vi "DFU_Foot_Data.vi"() -> ()   [LabVIEW 2016]
uses:
  <vilib>/Math Plots/3D Math Plots/3D Surface/3D Surface XCtrl/3D Surface.xctl
  <vilib>/Math Plots/3D Math Plots/3D Surface/3D Surface Datatype/Public/Plot Helper (Matrix).vi
  <vilib>/gmath/interp.llb/Interpolate 2D (2d X,Y).vi
  <vilib>/Math Plots/3D Math Plots/3D Surface/3D Surface Datatype/3D Surface Datatype.lvclass
  <vilib>/gmath/NI_Gmath.lvlib
panel:
  in  "Interpolation":i32(ring)=1 items=["nearest", "bilinear", "bicubic", "bicubic spline"]
  in  "Plot dT":u32=100
  out "Sample":i32
  out "Summed Plot":refnum<class "3D Plot Datatype.lvclass">[](xcontrol)
  out "Instantaneous Data":refnum<class "3D Plot Datatype.lvclass">[](xcontrol)
  out "Data Size":i32[](array[numeric])
  in  "Input Data Stream":dbl[][][](array[numeric])=array1101x8x8[70464 elements]
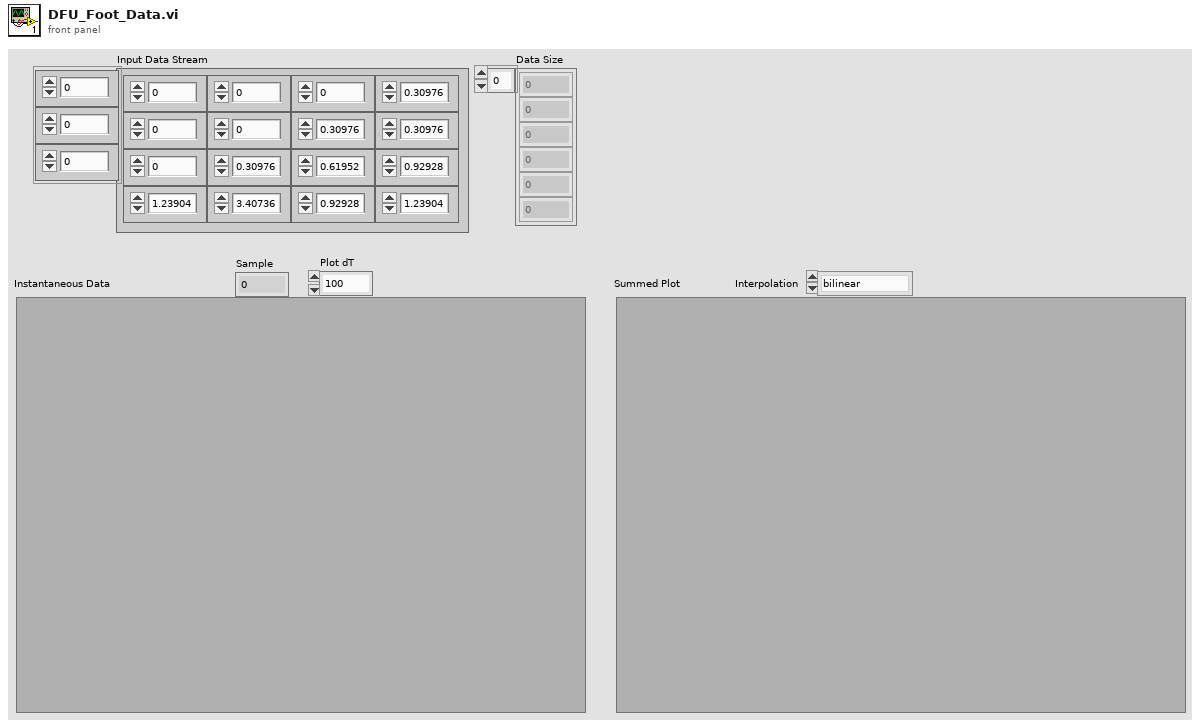
[diagram p1: front panel]
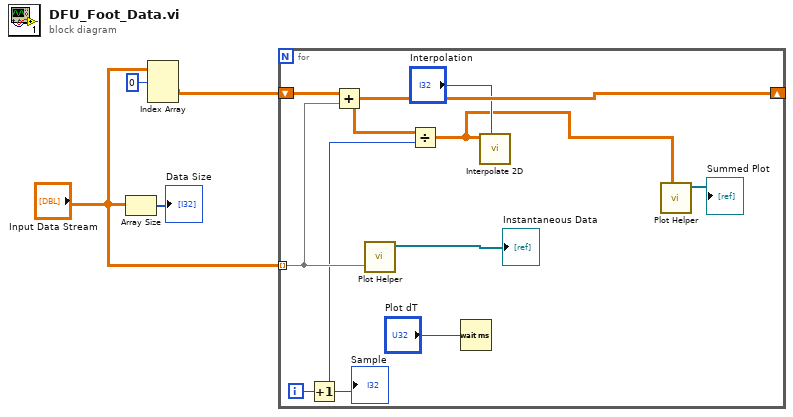
[diagram p0: block diagram]
diagram:
  n1 = Array Size(array="Input Data Stream") -> (size(s)=→"Data Size":i32[])
  n2 = Index Array(array="Input Data Stream", index (dim 0)=0 ("index (page)")) -> (element=w2:dbl[][])  [unwired: 2 in]
  n3 = for {
    tunnel: "Input Data Stream" -> [w10] mode=indexing
    shift-right: [w9] -> _
    shift-left: w2 -> [w11]
    i -> [w8]
    n4 = Increment(x=w8) -> (x+1=w7:i32)
    "Sample" <- w7
    n5 = Add(x=w11, y=w10) -> (x+y=w9:dbl[][])
    n6 = call-poly <vilib>:"Plot Helper.vi"("z matrix"=w10) -> ("3D Plot lvclass Array out"=→"Instantaneous Data":refnum<class "3D Plot Datatype.lvclass">[])  [unwired: 5 in, 5 out]
    n7 = Divide(x=w9, y=w7) -> (x/y=w5:dbl[][])
    n8 = Wait (ms)(milliseconds to wait="Plot dT") -> ()  [unwired: 1 out]
    n9 = call-poly <vilib>:"Interpolate 2D.vi"("method"="Interpolation", "Z"=w5) -> ()  [unwired: 6 in, 4 out]
    n10 = call-poly <vilib>:"Plot Helper.vi"("z matrix"=w5) -> ("3D Plot lvclass Array out"=→"Summed Plot":refnum<class "3D Plot Datatype.lvclass">[])  [unwired: 5 in, 5 out]
  }
